vi "SCE_load_charset_ROM.vi"(8 "error in":errorcluster, 10 "VIC-II D018":T1 {"video ram addr" format="%.0x"; "charset addr" format="%.0x"}, 11 "Charset ROM":path=path "D:/work/experimets/C64/rom/c64.bin") -> (0 "error out":errorcluster, 3 "char set":T2[](array[typedef]))   [LabVIEW 2018]
uses:
  SCE_character_bitmap.ctl
  SCE_VIC-II_reg_D018.ctl
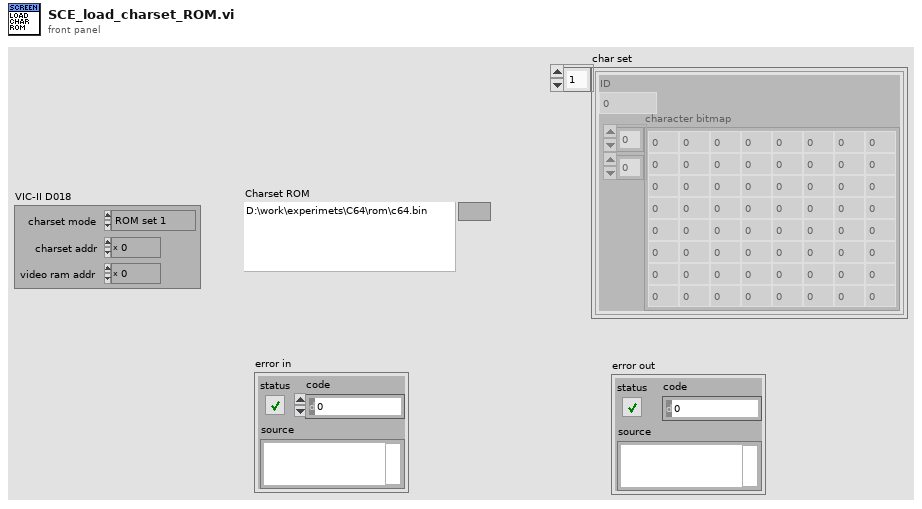
[diagram p1: front panel]
types:
  T1 = typedef "SCE_VIC-II_reg_D018.ctl" = cluster{"charset mode":enum16{"ROM set 1", "ROM set 2", "RAM"}, "charset addr":u16, "video ram addr":u16}
  T2 = typedef "SCE_character_bitmap.ctl" = cluster{"ID":i32, "character bitmap":u8[][]}
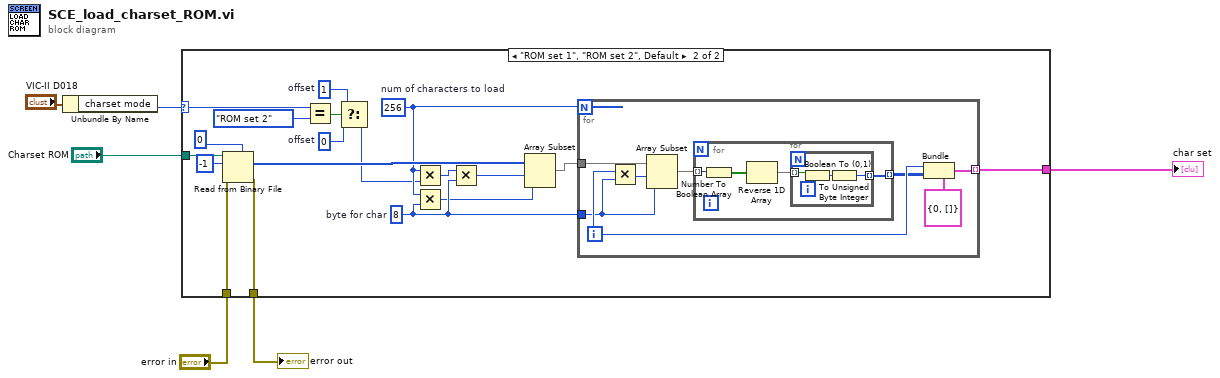
[diagram p0: block diagram]
diagram:
  n1 = Unbundle By Name("VIC-II D018") -> ("charset mode"=w1:enum16{"ROM set 1", "ROM set 2", "RAM"})
  n2 = case shown="\"ROM set 1\", \"ROM set 2\", Default" w1 {
    selector: w1 -> [_ w17]
    tunnel: "Charset ROM" -> [_ w24]
    tunnel: "error in" -> [w7 w20]
    tunnel: [w7 w19] -> w4
    tunnel: [_ w18] -> w3
    frame "RAM" {
    }
    frame "ROM set 1", "ROM set 2", Default {
      w13 = 0  # offset
      w14 = 1  # offset
      w11 = 8  # byte for char
      w21 = 256  # num of characters to load
      n3 = Read from Binary File(5:u8 0 ("Numeric"), 8:w20, 10:-1 ("count (1)"), 11:w24) -> (0:w19:errorcluster, 2:w23:u8[])  [unwired: 2 in, 2 out]
      n4 = Equal?(x=w17, y=enum16{"ROM set 1", "ROM set 2", "RAM"}."ROM set 2") -> (x = y?=w15:bool)
      n5 = Select(t=w14, s=w15, f=w13) -> (s? t:f=w12:i32)
      n6 = Multiply(x=w21, y=w12) -> (x*y=w10:i32)
      n7 = Multiply(x=w21, y=w11) -> (x*y=w8:i32)
      n8 = Multiply(x=w10, y=w11) -> (x*y=w9:i32)
      n9 = Array Subset(array=w23, index=w9, length=w8) -> (w22:u8[])
      n10 = for {
        N: w21 -> [_]
        tunnel: [w30] -> w18 mode=indexing
        tunnel: w22 -> [w34]
        tunnel: w11 -> [w27]
        i -> [w31]
        n11 = Multiply(x=w31, y=w27) -> (x*y=w32:i32)
        n12 = Array Subset(array=w34, index=w32, length=w27) -> (w33:u8[])
        n13 = for {
          tunnel: w33 -> [w37] mode=indexing
          tunnel: [w35] -> w29 mode=indexing
          n14 = Number To Boolean Array(number=w37) -> (Boolean array=w38:bool[])
          n15 = Reverse 1D Array(array=w38) -> (reversed array=w36:bool[])
          n16 = for {
            tunnel: w36 -> [w41] mode=indexing
            tunnel: [w39] -> w35 mode=indexing
            n17 = Boolean To (0,1)(Boolean=w41) -> (0, 1=w40:i16)
            n18 = To Unsigned Byte Integer(number=w40) -> (unsigned 8bit integer=w39:u8)
          }
        }
        n19 = Bundle(cluster=T2 {"ID"=0, "character bitmap"=[]}, "ID"=w31, "character bitmap"=w29) -> (w30:T2)
      }
    }
  }
  "error out" <- w4
  "char set" <- w3
